vi "Temperature Warnings.vi"() -> ()   [LabVIEW 2017]
doc: "This VI is used to determine the string to output to the weather station based on the current temperature and limit settings.\n\nInputs: Current Temperature (DBL), Minimum Temperature (DBL), and Maximum Temperature (DBL).\nOutputs: Warning Text (string) and Warning? (Boolean)."
uses:
  Weather Data.ctl
panel:
  out "Weather Data Out":T1={"Current Temperature"=0.0, "Max Temperature"=0.0, "Min Temperature"=0.0, "Warning?"=FALSE, "Warning Text"="No Warning", "Units"=""}
  in  "Weather Data In":T1={"Current Temperature"=0.0, "Max Temperature"=0.0, "Min Temperature"=0.0, "Warning?"=FALSE, "Warning Text"="No Warning", "Units"=""}
  out "Error Out":errorcluster
  in  "Error In":errorcluster
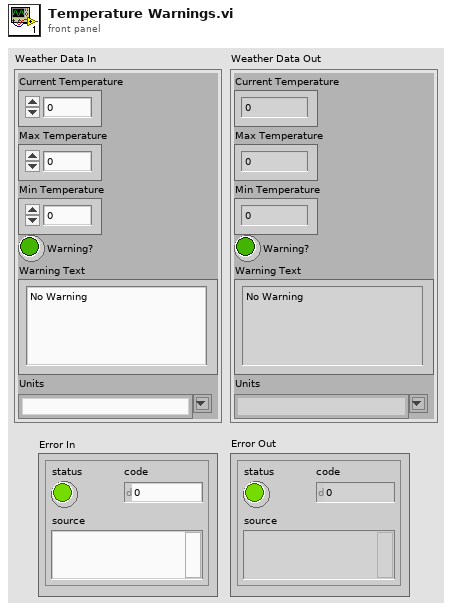
[diagram p1: front panel]
types:
  T1 = typedef "Weather Data.ctl" = cluster{"Current Temperature":dbl, "Max Temperature":dbl, "Min Temperature":dbl, "Warning?":bool, "Warning Text":string, "Units":string}
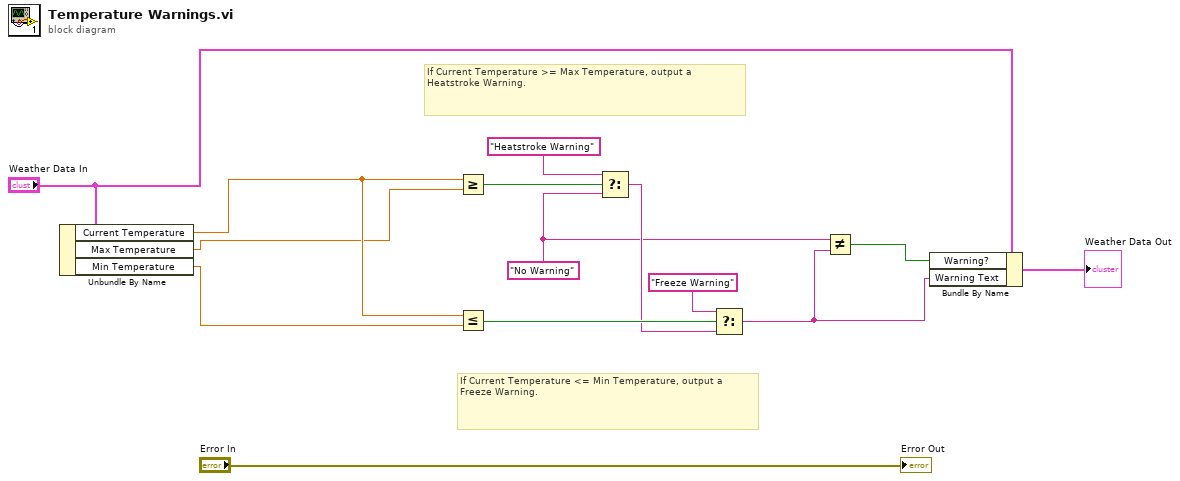
[diagram p0: block diagram]
diagram:
  w9 = "No Warning" ("f")
  # "If Current Temperature >= Max Temperature, output a Heatstroke Warning."
  # "If Current Temperature <= Min Temperature, output a Freeze Warning."
  n1 = Unbundle By Name("Weather Data In") -> ("Current Temperature"=w7:dbl, "Max Temperature"=w6:dbl, "Min Temperature"=w5:dbl)
  n2 = Greater Or Equal?(x=w7, y=w6) -> (x >= y?=w14:bool)
  n3 = Less Or Equal?(x=w7, y=w5) -> (x <= y?=w11:bool)
  n4 = Select(t="Heatstroke Warning", s=w14, f=w9) -> (s? t:f=w10:string)
  n5 = Select(t="Freeze Warning", s=w11, f=w10) -> (s? t:f=w1:string)
  n6 = Not Equal?(x=w9, y=w1) -> (x != y?=w2:bool)
  n7 = Bundle By Name(cluster="Weather Data In", "Warning?"=w2, "Warning Text"=w1) -> (→"Weather Data Out":T1)
  "Error Out" <- "Error In"
